vi "trafic light (2).vi"() -> ()   [LabVIEW 2021]
panel:
  in  "Yellow time 4":dbl
  in  "Green time 2":dbl
  in  "Yellow time 3":dbl
  in  "Red time 2":dbl
  in  "?":bool
  out "Time 2":dbl
  out "Green 2":bool
  out "Yellow 2":bool
  out "Red 2":bool
  in  "Yellow time 2":dbl
  out "Time":dbl
  out "Green":bool
  in  "Green time":dbl
  in  "Yellow time":dbl
  in  "Red time":dbl
  in  "?":bool
  out "Yellow":bool
  out "Red":bool
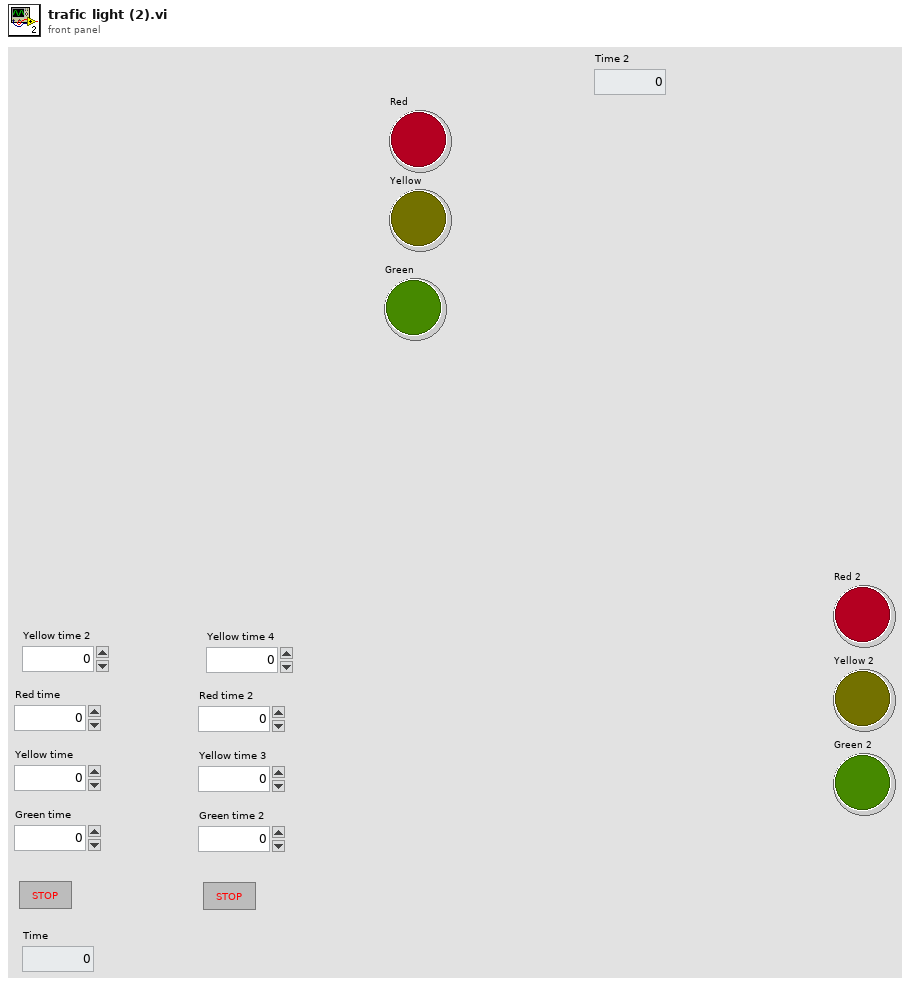
[diagram p1: front panel]
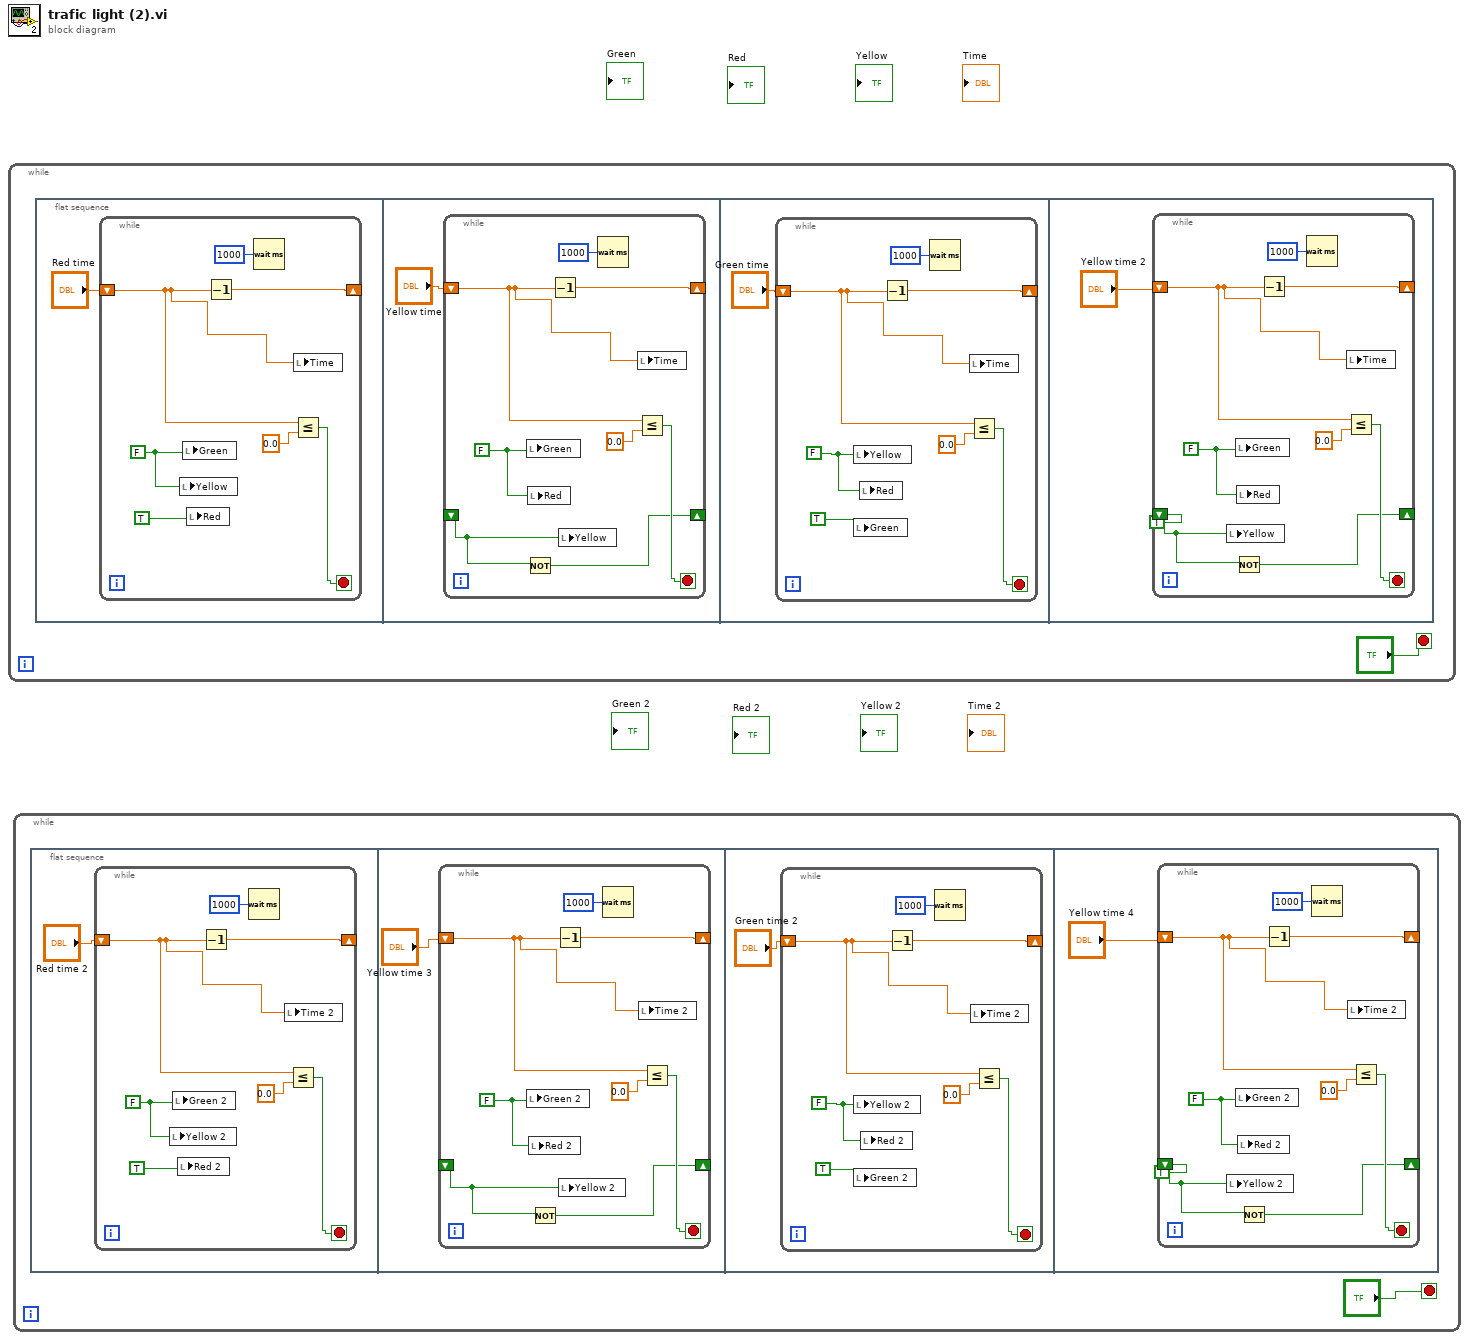
[diagram p0: block diagram]
diagram:
  n1 = while {
    stop <- "?" stop-if-true
    n2 = flat-sequence {
      frame #0 {
        n3 = while {
          shift-right: [w7] -> _
          shift-left: "Red time" -> [w6]
          stop <- w4 stop-if-true
          w9 = FALSE
          n4 = local write "Yellow"(w9) -> ()
          n5 = local write "Green"(w9) -> ()
          n6 = local write "Red"(TRUE) -> ()
          n7 = Decrement(x=w6) -> (x-1=w7:dbl)
          n8 = Wait (ms)(milliseconds to wait=u32 1000) -> ()  [unwired: 1 out]
          n9 = Less Or Equal?(x=w6, y=0.0) -> (x <= y?=w4:bool)
          n10 = local write "Time"(w6) -> ()
        }
      }
      frame #1 {
        n11 = while {
          shift-right: [w18] -> _
          shift-left: "Yellow time" -> [w17]
          shift-right: [w12] -> _
          shift-left: _ -> [w11]
          stop <- w15 stop-if-true
          w13 = FALSE
          n12 = Not(x=w11) -> (.not. x?=w12:bool)
          n13 = local write "Green"(w13) -> ()
          n14 = local write "Red"(w13) -> ()
          n15 = Decrement(x=w17) -> (x-1=w18:dbl)
          n16 = local write "Yellow"(w11) -> ()
          n17 = Wait (ms)(milliseconds to wait=u32 1000) -> ()  [unwired: 1 out]
          n18 = Less Or Equal?(x=w17, y=0.0) -> (x <= y?=w15:bool)
          n19 = local write "Time"(w17) -> ()
        }
      }
      frame #2 {
        n20 = while {
          shift-right: [w26] -> _
          shift-left: "Green time" -> [w25]
          stop <- w23 stop-if-true
          w21 = FALSE
          n21 = local write "Yellow"(w21) -> ()
          n22 = local write "Green"(TRUE) -> ()
          n23 = local write "Red"(w21) -> ()
          n24 = Decrement(x=w25) -> (x-1=w26:dbl)
          n25 = Wait (ms)(milliseconds to wait=u32 1000) -> ()  [unwired: 1 out]
          n26 = Less Or Equal?(x=w25, y=0.0) -> (x <= y?=w23:bool)
          n27 = local write "Time"(w25) -> ()
        }
      }
      frame #3 {
        n28 = while {
          shift-right: [w36] -> _
          shift-left: "Yellow time 2" -> [w35]
          shift-right: [w30] -> _
          shift-left: TRUE -> [w29]
          stop <- w33 stop-if-true
          w31 = FALSE
          n29 = local write "Yellow"(w29) -> ()
          n30 = Not(x=w29) -> (.not. x?=w30:bool)
          n31 = local write "Green"(w31) -> ()
          n32 = local write "Red"(w31) -> ()
          n33 = Decrement(x=w35) -> (x-1=w36:dbl)
          n34 = Wait (ms)(milliseconds to wait=u32 1000) -> ()  [unwired: 1 out]
          n35 = Less Or Equal?(x=w35, y=0.0) -> (x <= y?=w33:bool)
          n36 = local write "Time"(w35) -> ()
        }
      }
    }
  }
  n37 = while {
    stop <- "?" stop-if-true
    n38 = flat-sequence {
      frame #0 {
        n39 = while {
          shift-right: [w43] -> _
          shift-left: "Red time 2" -> [w42]
          stop <- w40 stop-if-true
          w45 = FALSE
          n40 = local write "Yellow 2"(w45) -> ()
          n41 = local write "Green 2"(w45) -> ()
          n42 = local write "Red 2"(TRUE) -> ()
          n43 = Decrement(x=w42) -> (x-1=w43:dbl)
          n44 = Wait (ms)(milliseconds to wait=u32 1000) -> ()  [unwired: 1 out]
          n45 = local write "Time 2"(w42) -> ()
          n46 = Less Or Equal?(x=w42, y=0.0) -> (x <= y?=w40:bool)
        }
      }
      frame #1 {
        n47 = while {
          shift-right: [w54] -> _
          shift-left: "Yellow time 3" -> [w53]
          shift-right: [w48] -> _
          shift-left: _ -> [w47]
          stop <- w51 stop-if-true
          w49 = FALSE
          n48 = local write "Green 2"(w49) -> ()
          n49 = local write "Red 2"(w49) -> ()
          n50 = Not(x=w47) -> (.not. x?=w48:bool)
          n51 = Decrement(x=w53) -> (x-1=w54:dbl)
          n52 = local write "Yellow 2"(w47) -> ()
          n53 = Wait (ms)(milliseconds to wait=u32 1000) -> ()  [unwired: 1 out]
          n54 = local write "Time 2"(w53) -> ()
          n55 = Less Or Equal?(x=w53, y=0.0) -> (x <= y?=w51:bool)
        }
      }
      frame #2 {
        n56 = while {
          shift-right: [w62] -> _
          shift-left: "Green time 2" -> [w61]
          stop <- w59 stop-if-true
          w57 = FALSE
          n57 = local write "Yellow 2"(w57) -> ()
          n58 = local write "Green 2"(TRUE) -> ()
          n59 = local write "Red 2"(w57) -> ()
          n60 = Decrement(x=w61) -> (x-1=w62:dbl)
          n61 = Wait (ms)(milliseconds to wait=u32 1000) -> ()  [unwired: 1 out]
          n62 = local write "Time 2"(w61) -> ()
          n63 = Less Or Equal?(x=w61, y=0.0) -> (x <= y?=w59:bool)
        }
      }
      frame #3 {
        n64 = while {
          shift-right: [w72] -> _
          shift-left: "Yellow time 4" -> [w71]
          shift-right: [w66] -> _
          shift-left: TRUE -> [w65]
          stop <- w69 stop-if-true
          w67 = FALSE
          n65 = local write "Yellow 2"(w65) -> ()
          n66 = local write "Green 2"(w67) -> ()
          n67 = local write "Red 2"(w67) -> ()
          n68 = Not(x=w65) -> (.not. x?=w66:bool)
          n69 = Decrement(x=w71) -> (x-1=w72:dbl)
          n70 = Wait (ms)(milliseconds to wait=u32 1000) -> ()  [unwired: 1 out]
          n71 = local write "Time 2"(w71) -> ()
          n72 = Less Or Equal?(x=w71, y=0.0) -> (x <= y?=w69:bool)
        }
      }
    }
  }
